vi "GF_AgilentTestChannelRead.vi"() -> ()   [LabVIEW 2009]
panel:
  out "Token Array 2":cluster{"Name":string, "Value":string}[](array[cluster])
  in  "Timeout (10000 ms)":u32=10000
  in  "Source (0: Channel 1)":u16(ring) items=["Channel 1", "Channel 2", "Channel 3", "Channel 4", "Math"]
  out "error out":errorcluster
  in  "error in (no error)":errorcluster
  in  "VISA resource name In":refnum<visa-resource-name>
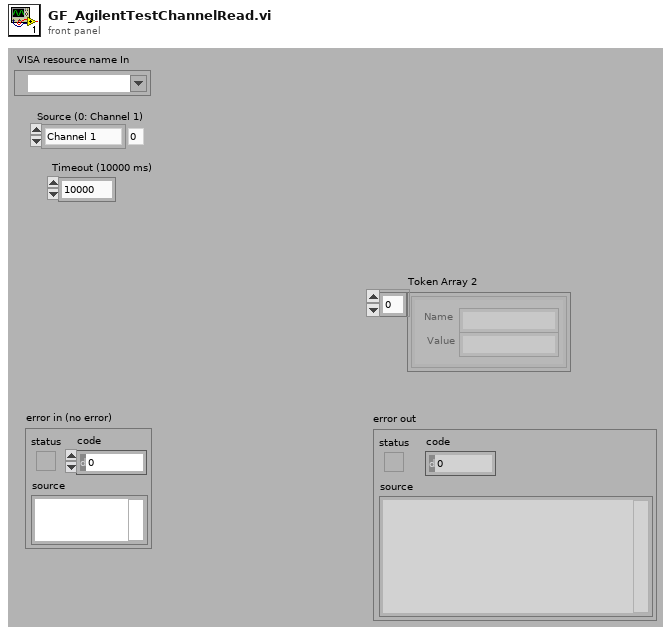
[diagram p1: front panel]
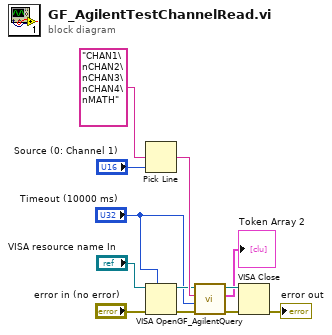
[diagram p0: block diagram]
diagram:
  n1 = Pick Line(multi-line string="CHAN1\nCHAN2\nCHAN3\nCHAN4\nMATH", line index="Source (0: Channel 1)") -> (output string=w5:string)  [unwired: 1 in]
  n2 = VISA Open(timeout (0)="Timeout (10000 ms)", error in (no error)="error in (no error)", VISA resource name="VISA resource name In") -> (VISA resource name=w4:refnum<visa-resource-name>, error out=w3:errorcluster)  [unwired: 2 in]
  n3 = call "GF_AgilentQuery.vi"("error in (no error)"=w3, "Timeout"="Timeout (10000 ms)", "Query"=w5, "Session In"=w4) -> ("error out"=w6:errorcluster, "Token Array 2"=→"Token Array 2":cluster{"Name":string, "Value":string}[], "Session out"=w7:refnum<visa-resource-name>)  [unwired: 4 in]
  n4 = VISA Close(VISA resource name=w7, error in (no error)=w6) -> (error out=→"error out":errorcluster)
